vi "ProgressDataAnalyzer.vi"() -> ()   [LabVIEW 2020]
uses:
  <vilib>/Skyline/Tag/Shared/typedefs/DataType.ctl
  <vilib>/Skyline/Configuration/Configuration HTTP_class/NI Skyline Configuration HTTP.lvclass/NI Skyline Configuration HTTP.ctl
  <vilib>/Skyline/Configuration/Configuration HTTP_class/Open Configuration HTTP.vi
  <vilib>/Skyline/Configuration/HTTP/Open Configuration (Desktop).vi
  <vilib>/Skyline/Tag/Wrapper/Wrapper HTTP_class/Open Tag HTTP.vi
  <vilib>/Skyline/Tag/Wrapper/Wrapper_class/Write Tag (DBL).vi
  <vilib>/Skyline/Tag/Wrapper/Wrapper_class/Delete Tag (Single).vi
  <vilib>/Skyline/Configuration/Configuration HTTP_class/NI Skyline Configuration HTTP.lvclass
  <vilib>/Skyline/Configuration/Configuration_class/NI Skyline Configuration.lvclass
  <vilib>/Skyline/Tag/Wrapper/Wrapper_class/NI Skyline Tag.lvclass
  <vilib>/Skyline/Tag/Wrapper/Wrapper HTTP_class/NI Skyline Tag HTTP.lvclass
  <vilib>/Skyline/Tag/Shared/NI Skyline Tag.lvlib
panel:
  in  "stop":bool
  out "Progress":u8(slide) scale=0.0..100.0
  in  "Test Drive Distance":dbl
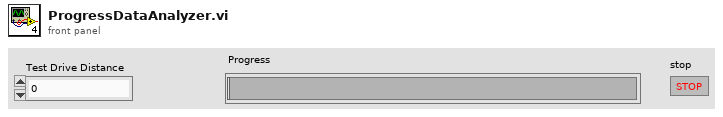
[diagram p1: front panel]
types:
  T1 = typedef "NI Skyline Tag.lvlib/DataType.ctl" = enum32{"Double", "I32", "String", "Boolean", "U64", "Timestamp"}
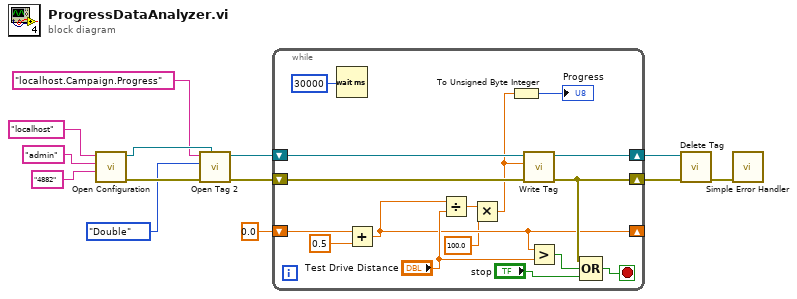
[diagram p0: block diagram]
diagram:
  n1 = call-poly <vilib>:"Open Configuration.vi"("password"="4882", "username"="admin", "server url"="localhost") -> ("error out"=w12:errorcluster, "configuration"=w13:refnum<class "NI Skyline Configuration HTTP.lvclass">)  [unwired: 7 in]
  n2 = call-poly <vilib>:"Open Tag 2.vi"("configuration"=w13, "error in (no error)"=w12, "Data Type"=DataType."Double", "path"="localhost.Campaign.Progress") -> ("error out"=w5:errorcluster, "tag"=w6:refnum<class "NI Skyline Tag.lvclass">)  [unwired: 6 in]
  n3 = while {
    shift-right: [w27] -> w4
    shift-left: w6 -> [w29]
    shift-right: [w24] -> w3
    shift-left: w5 -> [w28]
    shift-right: [w19] -> _
    shift-left: 0.0 -> [w22]
    stop <- w25 stop-if-true
    n4 = Wait (ms)(milliseconds to wait=u32 30000) -> ()  [unwired: 1 out]
    n5 = Add(x=w22, y=0.5) -> (x+y=w19:dbl)
    n6 = Divide(x=w19, y="Test Drive Distance") -> (x/y=w18:dbl)
    n7 = Multiply(x=w18, y=100.0) -> (x*y=w16:dbl)
    n8 = To Unsigned Byte Integer(number=w16) -> (unsigned 8bit integer=→"Progress":u8)
    n9 = call-poly <vilib>:"Write Tag.vi"("error in (no error)"=w28, "value"=w16, "tag in"=w29) -> ("error out"=w24:errorcluster, "tag out"=w27:refnum<class "NI Skyline Tag.lvclass">)  [unwired: 7 in]
    n10 = Greater?(x=w19, y="Test Drive Distance") -> (0:w21:bool)
    n11 = Compound Arithmetic op=OR(w24, w21, "stop") -> (w25:bool)
  }
  n12 = call-poly <vilib>:"Delete Tag.vi"("error in (no error)"=w3, "tag"=w4) -> ("error out"=w1:errorcluster)  [unwired: 9 in]
  n13 = call <vilib>:"Simple Error Handler.vi"("error in (no error)"=w1) -> ()  [unwired: 4 in, 5 out]
